vi "performanceCalc.vi"(0 "errors":dbl[](array[numeric]), 1 "init":bool, 2 "windowLength":dbl, 5 "pckTotalTrack":dbl[](array[numeric]), 7 "state":dbl[](array[numeric]), 9 "pckSuccess":dbl, 11 "pckTotal":dbl, 12 "delay":dbl) -> (4 "errorsOut":dbl[](array[numeric]), 6 "pckTotalTrackOut":dbl[](array[numeric]), 8 "prevState":dbl[](array[numeric]))   [LabVIEW 2009]
uses:
  <vilib>/imath/engines/lvmath2/RunTimeEngine/ErrorHandling/NIMS_Finalize Error.vi
  <vilib>/imath/engines/lvmath2/RunTimeEngine/Parser/MC_Version.vi
  <vilib>/imathl/engines/lvmath/Functions/Error Handling/Create Error.vi
  <vilib>/imath/engines/lvmath2/RunTimeEngine/VariableToken/Read/NIMS_Get Elements - RV(_) - Check.vi
  <instcachedir>/0/NIMS_Get Elements - RV(_) - Check_60F12861D0564803969A5D0D0D1716CD.lvgen/NIMS_Get Elements - RV(_) - Check_60F12861D0564803969A5D0D0D1716CD_000.vi
  <vilib>/imath/engines/lvmath2/RunTimeEngine/NodeEndStatement/NIMS_NodeEndStatement_Output.vi
  <instcachedir>/0/NIMS_NodeEndStatement_Output_B70DDD75627E4997AAE11E9955EDAA25.lvgen/NIMS_NodeEndStatement_Output_B70DDD75627E4997AAE11E9955EDAA25_001.vi
  <instcachedir>/0/NIMS_NodeEndStatement_Output_B70DDD75627E4997AAE11E9955EDAA25.lvgen/NIMS_NodeEndStatement_Output_B70DDD75627E4997AAE11E9955EDAA25_000.vi
  <vilib>/imath/engines/lvmath/Functions/Error Handling/MergeErrorsWrapper.vi
  <vilib>/imath/engines/lvmath2/RunTimeEngine/BuiltInFunctions/mod/NIMS_mod_no_size_check.vi
  <instcachedir>/0/NIMS_mod_no_size_check_666FA8FF03DD4BACB539E38A2DCFE11D.lvgen/NIMS_mod_no_size_check_666FA8FF03DD4BACB539E38A2DCFE11D_000.vi
  <vilib>/imath/engines/lvmath2/RunTimeEngine/ReplaceToken/NIMS_Replace - V(S)=S.vi
  <instcachedir>/0/NIMS_Replace - V(S)=S_670A9E0533664C1D848C8E58B3321B6A.lvgen/NIMS_Replace - V(S)=S_670A9E0533664C1D848C8E58B3321B6A_000.vi
  <vilib>/imath/engines/lvmath2/RunTimeEngine/ReplaceToken/NIMS_Replace - Size Check _(_)=S.vi
  <instcachedir>/0/NIMS_Replace - Size Check _(_)=S_8596181D73404097BAB9CBB006194BB0.lvgen/NIMS_Replace - Size Check _(_)=S_8596181D73404097BAB9CBB006194BB0_000.vi
  <vilib>/imath/engines/lvmath2/RunTimeEngine/ReplaceToken/NIMS_Replace - Check(_) Linear.vi
  <instcachedir>/0/NIMS_Replace - Check(_) Linear_ADCB184354B04941957EC3DDF82F7E42.lvgen/NIMS_Replace - Check(_) Linear_ADCB184354B04941957EC3DDF82F7E42_000.vi
  <vilib>/imath/engines/lvmath2/RunTimeEngine/VariableToken/Read/NIMS_Get Elements - RV(_) - Check(_).vi
  <instcachedir>/0/NIMS_Get Elements - RV(_) - Check(_)_82E0F2002B964B63A6FF4E3708911C3C.lvgen/NIMS_Get Elements - RV(_) - Check(_)_82E0F2002B964B63A6FF4E3708911C3C_000.vi
  <vilib>/imath/engines/lvmath2/RunTimeEngine/BuiltInFunctions/sum/NIMS_sum(GV).vi
  <instcachedir>/0/NIMS_sum(GV)_6582ACC3CFD94C22B1CA3BD4A8C5E9ED.lvgen/NIMS_sum(GV)_6582ACC3CFD94C22B1CA3BD4A8C5E9ED_000.vi
  <vilib>/imath/engines/lvmath2/RunTimeEngine/ReplaceToken/NIMS_Replace - Check Linear.vi
  <instcachedir>/0/NIMS_Replace - Check Linear_9243CBB174894FF6977027453DA6955E.lvgen/NIMS_Replace - Check Linear_9243CBB174894FF6977027453DA6955E_000.vi
panel:
  out "interSampling":dbl
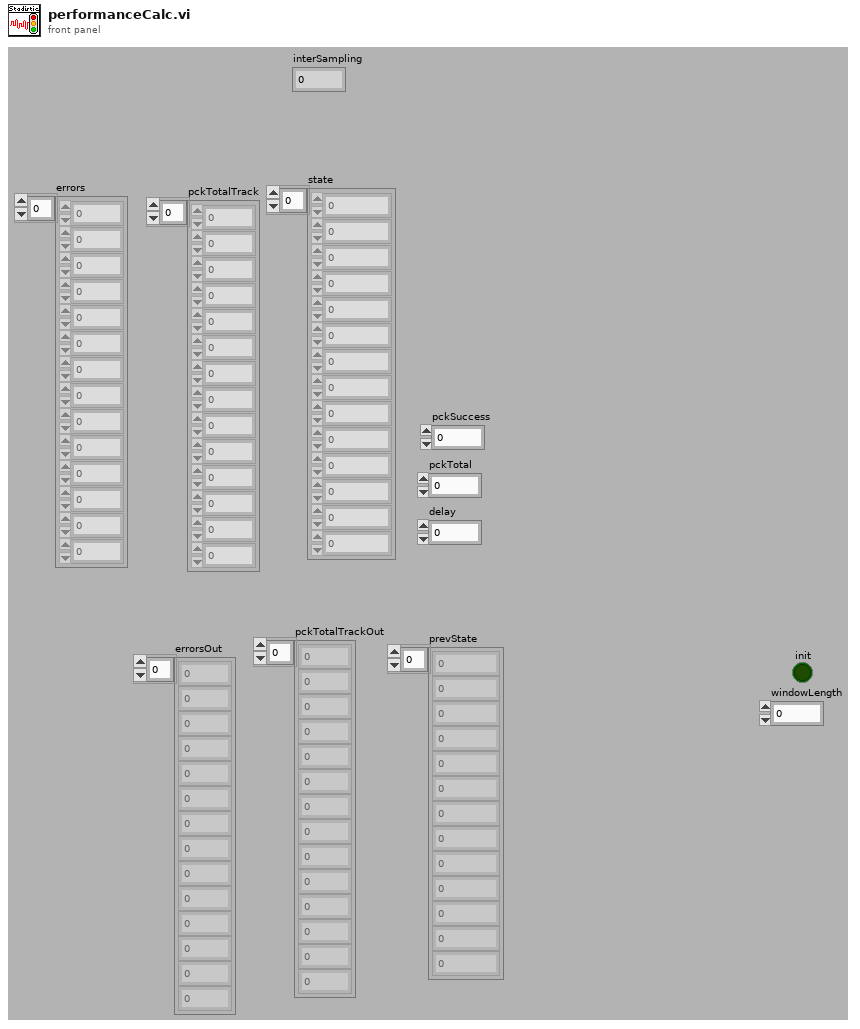
[diagram p1: front panel]
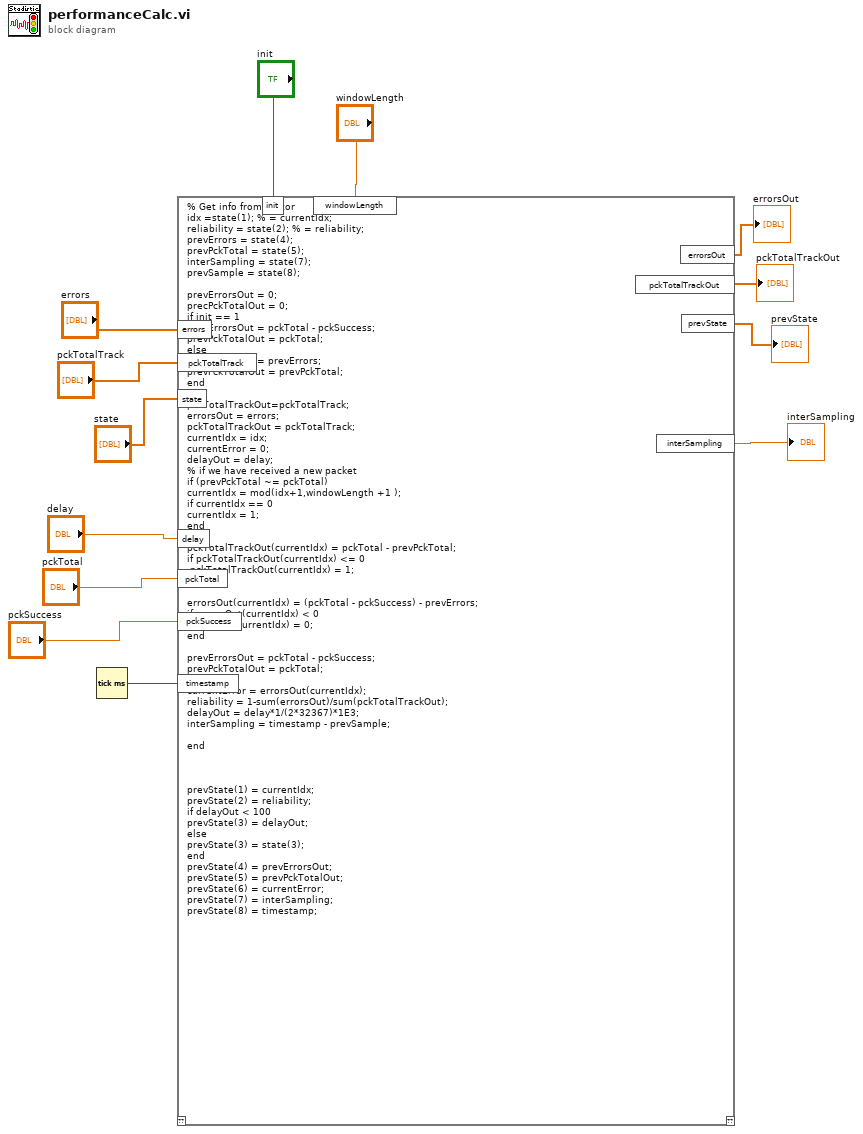
[diagram p0: block diagram]
diagram:
  n1 = Tick Count (ms)() -> (millisecond timer value=w2:u32)
  n2 = mathscript code="% Get info from vector\nidx =state(1); % = currentIdx;\nreliability = state(2); % = reliability;\nprevErrors = state(4);\nprevPckTotal = state(5);\ninterSampling = state(7);\nprevSample = state(8);\n\nprevErrorsOut = 0;\nprecPckTotalOut = 0;\nif init == 1\nprevErrorsOut = pckTotal - pckSuccess;\nprevPckTotalOut = pckTotal;\nelse\nprevErrorsOut = prevErrors;\nprevPckTotalOut = prevPckTotal;\nend\n\npckTotalTrackOut=pckTotalTrack;\nerrorsOut = errors;\npckTotalTrackOut = pckTotalTrack;\ncurrentIdx = idx;\ncurrentError = 0;\ndelayOut = delay;\n% if we have received a new packet\nif (prevPckTotal ~= pckTotal)\ncurrentIdx = mod(idx+1,windowLength +1 );\nif currentIdx == 0\ncurrentIdx = 1;\nend\n\npckTotalTrackOut(currentIdx) = pckTotal - prevPckTotal;\nif pckTotalTrackOut(currentIdx) <= 0\n pckTotalTrackOut(currentIdx) = 1;\nend\n\nerrorsOut(currentIdx) = (pckTotal - pckSuccess) - prevErrors;\nif errorsOut(currentIdx) < 0\nerrorsOut(currentIdx) = 0;\nend\n\nprevErrorsOut = pckTotal - pckSuccess;\nprevPckTotalOut = pckTotal;\n\ncurrentError = errorsOut(currentIdx);\nreliability = 1-sum(errorsOut)/sum(pckTotalTrackOut);\ndelayOut = delay*1/(2*32367)*1E3;\ninterSampling = timestamp - prevSample;\n\nend\n\n\n\nprevState(1) = currentIdx;\nprevState(2) = reliability;\nif delayOut < 100\nprevState(3) = delayOut;\nelse\nprevState(3) = state(3);\nend\nprevState(4) = prevErrorsOut;\nprevState(5) = prevPckTotalOut;\nprevState(6) = currentError;\nprevState(7) = interSampling;\nprevState(8) = timestamp;"("pckSuccess"="pckSuccess", "pckTotal"="pckTotal", "delay"="delay", "errors"="errors", "pckTotalTrack"="pckTotalTrack", "windowLength"="windowLength", "init"="init", "state"="state", "timestamp"=w2) -> ("errorsOut"=→"errorsOut":dbl[], "pckTotalTrackOut"=→"pckTotalTrackOut":dbl[], "prevState"=→"prevState":dbl[], "interSampling"=→"interSampling":dbl)  [unwired: 1 in, 1 out]
